vi "Position Play Video Button.vi"(8 "error in (no error)":errorcluster, 10 "Side tab":refnum<vi>, 11 "Button Ref":refnum<vi>) -> (0 "error out":errorcluster)   [LabVIEW 2014]
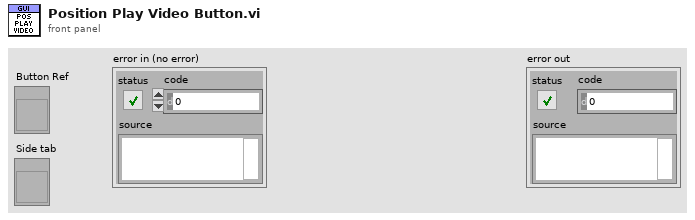
[diagram p1: front panel]
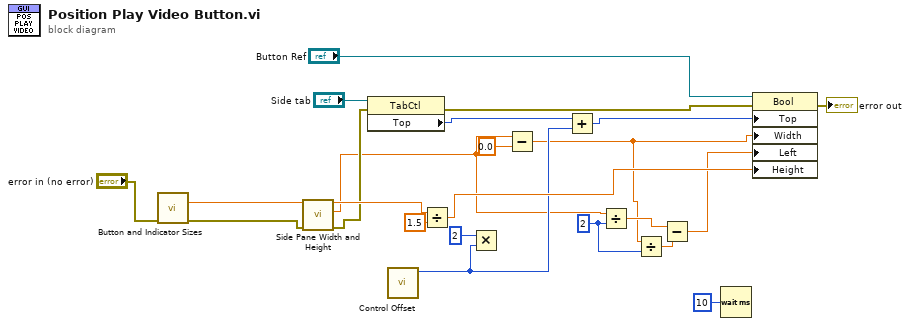
[diagram p0: block diagram]
diagram:
  w9 = u32 2 ("y")
  n1 = call "Button and Indicator Sizes.vi"("error in (no error)"="error in (no error)") -> ("Button Height"=w17:dbl, "error out"=w4:errorcluster)  [unwired: 10 in, 3 out]
  n2 = call "Side Pane Width and Height.vi"("error in (no error)"=w4) -> ("error out"=w3:errorcluster, "Width"=w2:dbl)  [unwired: 8 in, 1 out]
  n3 = property class="TabCtl"(reference="Side tab", error in=w3) -> (error out=w21:errorcluster, "Top"=w14:i32)  [unwired: 1 out]
  n4 = call "Control Offset.vi"() -> ("Offset From Tab Edge in (px)"=w12:i32)  [unwired: 11 in]
  n5 = Divide(x=w17, y=1.5) -> (x/y=w15:dbl)
  n6 = Multiply(x=2, y=w12) -> ()  [unwired: 1 out]
  n7 = Subtract(x=w2, y=0.0) -> (x-y=w7:dbl)
  n8 = Add(x=w14, y=w12) -> (x+y=w13:i32)
  n9 = Divide(x=w2, y=w9) -> (x/y=w8:dbl)
  n10 = Divide(x=w7, y=w9) -> (x/y=w10:dbl)
  n11 = Subtract(x=w8, y=w10) -> (x-y=w6:dbl)
  n12 = Wait (ms)(milliseconds to wait=u32 10) -> ()  [unwired: 1 out]
  n13 = property class="Bool"(reference="Button Ref", error in=w21, "Top"=w13, "Width"=w7, "Left"=w6, "Height"=w15) -> (error out=→"error out":errorcluster)  [unwired: 1 out]
